vi "excelrowconcat.vi"() -> ()   [LabVIEW 2020]
uses:
  <vilib>/addons/_office/excel.llb/Excel Get Data ([dbl]).vi
  <vilib>/Utility/file.llb/Write To Spreadsheet File (DBL).vi
  <vilib>/Utility/NIReport.llb/NI_report.lvclass
  <vilib>/Utility/NIReport.llb/Excel/NI_Excel.lvclass
  <vilib>/addons/_office/NI_ReportGenerationToolkit.lvlib
panel:
  out "# Columns":i32
  out "# Rows":i32
  in  "Excel._Worksheet":refnum<k7>
  in  "Excel._Application":refnum<k7>
  out "Stack Col":ext[](array[numeric]) format="%#_6e"
  out "Selected Column":ext[](array[numeric])=[3.90764143958222e-05, 7.61822884669527e-05, 0.000114766080514528, 0.000154096182086505, 0.000194036736502312, 0.000211308521102183, 0.000244270893745124, 0.000280356936855242, 0.000316674588248134, 0.000346021261066198, 0.000431595311965793, 0.000475546228699386, 0.00051031302427873, 0.000549825024791062, 0.000611612165812403, 0.000633780786301941, 0.000619862112216651, 0.000508421915583313, 0.000282114429865032, 0.000305013061733916, 0.000323792832205072, 0.000337357050739229, 0.000354817893821746, 0.00036767779965885, 0.0004547196731437, 0.000476125016575679, 0.000460526207461953, 0.000503468560054898, 0.000534854829311371, 0.000561434135306627, 0.000575784360989928, 0.000602852320298553, 0.00058649032143876, 0.000528524222318083, 0.00047412229469046, 0.000426320446422324, 0.000394057540688664, 0.00035078008659184, 0.000306837755488232, 0.00027094132383354, 0.000238187931245193, 0.000209086530958302, 0.000183560623554513, 0.000159952367539518, 0.000138665272970684, 0.000119993324915413, 0.000103645805211272, 8.89317743713036e-05, 7.6019176049158e-05, 6.45195468678139e-05, 5.44001304660924e-05, 4.54942346550524e-05, 3.67294742318336e-05, 3.00935225823196e-05, 2.41571360675152e-05, 1.92496518138796e-05, 1.50192872752086e-05, 1.14403846964706e-05, 8.30091448733583e-06, 5.93545382798766e-06, 4.11274368161685e-06, 2.75384900305653e-06, 1.63597394475801e-06, 7.48674267470051e-07, 1.28115464903544e-08] format="%#_6e"
  in  "precission":string="6"
  in  "Destination path for cutting rows":path=path "C:/Users/lab user/Desktop/cm/New folder (2)"
  in  "row cut file name (no extension)":string="resultd9.xls"
  out "selected row":ext[](array[numeric])=[5.0, 14.0, 24.0, 34.887542] format="%#_6e"
  in  "Select Row Number (1,2,)":string="1,3,5"
  out "Total Selected Row":i32=3
  in  "Select Excel file":path=path "C:/Users/lab user/Desktop/cm/New folder (2)/D9.xls"
  out "Output Added row":ext[][](array[numeric])=[[1.0, 10.45566, 20.0, 30.0], [3.0, 12.0, 22.8765, 32.0], [5.0, 14.0, 24.0, 34.887542]] format="%#_6e"
  out "Sheet Values":ext[][](array[numeric])=[[1.0, 10.45566, 20.0, 30.0], [2.0, 11.0, 21.0, 31.0], [3.0, 12.0, 22.8765, 32.0], [4.0, 13.0, 23.0, 33.0], [5.0, 14.0, 24.0, 34.887542], [6.0, 15.0, 25.0, 35.0], [7.0, 16.0, 26.0, 36.0], [8.0, 17.0, 27.0, 37.0], [9.0, 18.0, 28.0, 38.0], [10.0, 19.0, 29.0, 39.0], [11.0, 20.0, 30.0, 40.0], [12.0, 21.0, 31.0, 41.0], [13.0, 22.0, 32.0, 42.0], [14.0, 23.0, 33.0, 43.0], [15.0, 24.0, 34.0, 44.0], [16.0, 25.0, 35.0, 45.0], [17.0, 26.0, 36.0, 46.0], [18.0, 27.0, 37.0, 47.0], [19.0, 28.0, 38.0, 48.0], [20.0, 29.0, 39.0, 49.0], [21.0, 30.0, 40.0, 50.0], [22.0, 31.0, 41.0, 51.0], [23.0, 32.0, 42.0, 52.0]] format="%_6e"
  # "_single column output will be save in same directory\nrow cut file name_single_col.xls"
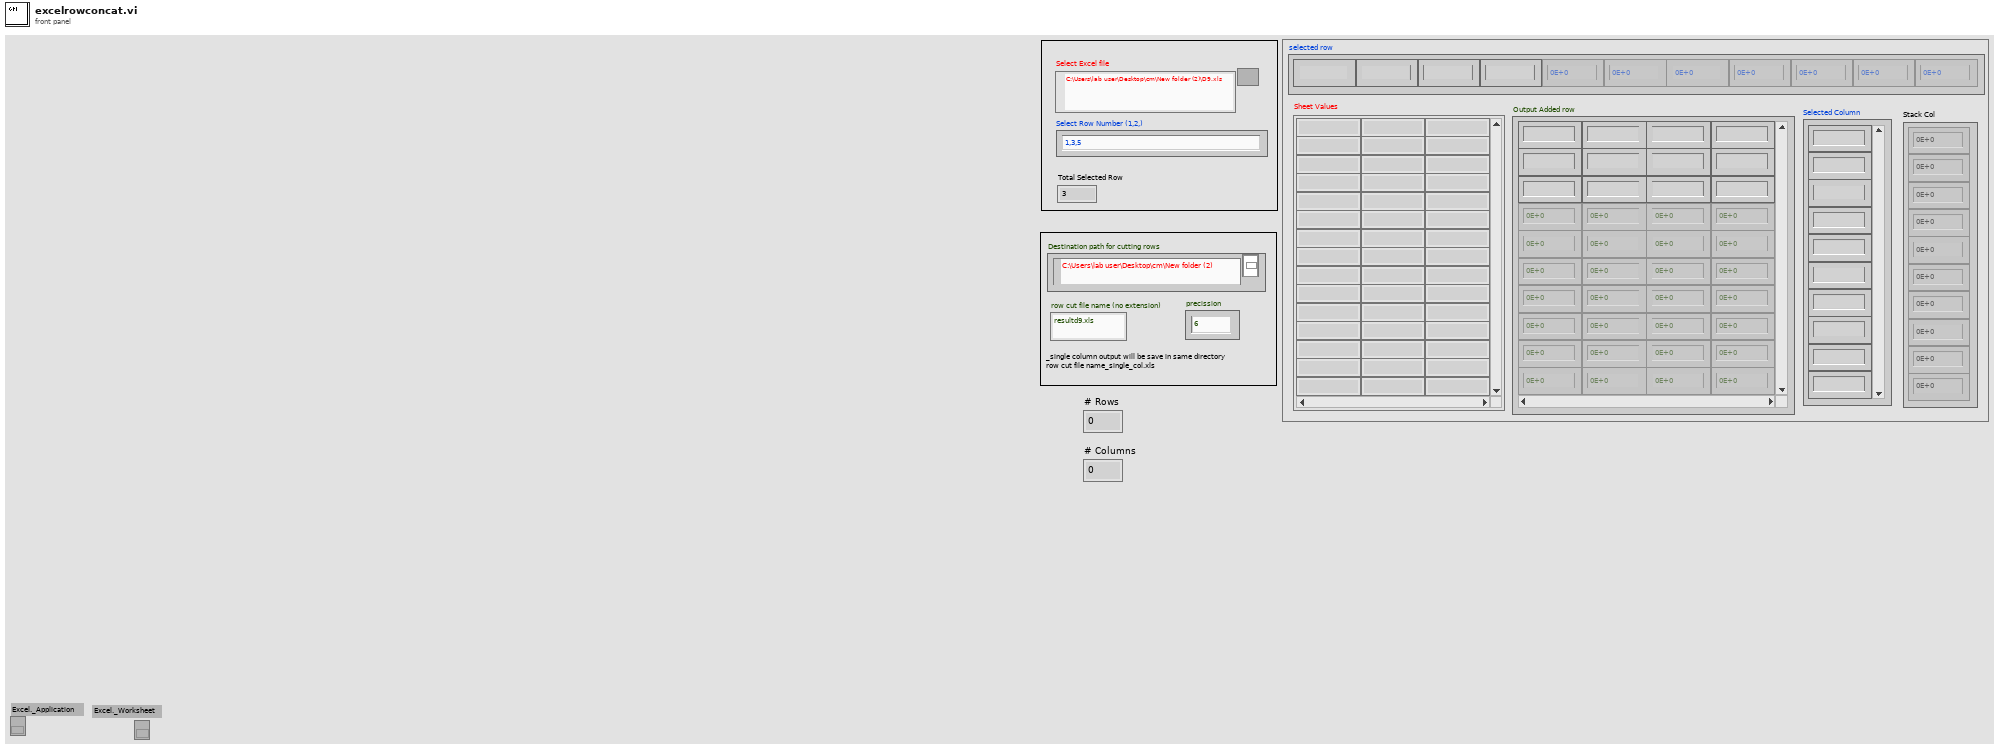
[diagram p1: front panel]
types:
  T1 = enum16{"Standard Report", "HTML", "Word", "Excel"}
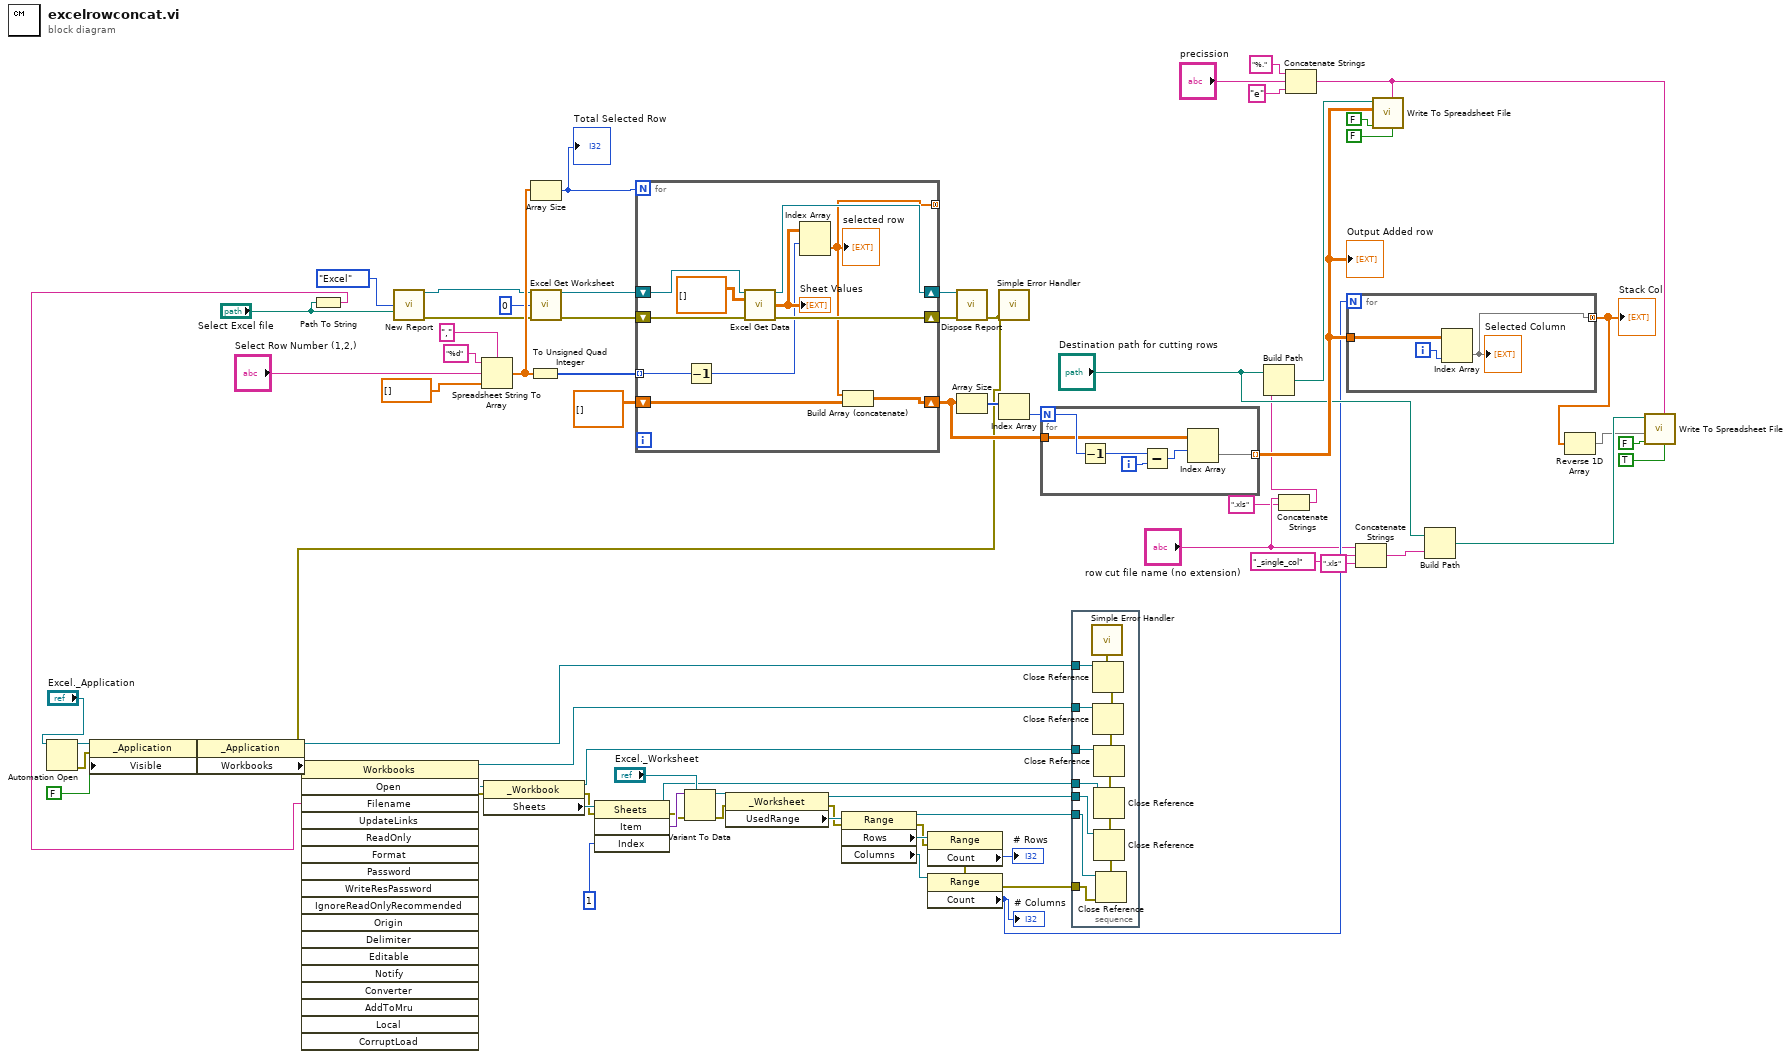
[diagram p0: block diagram]
diagram:
  n1 = Automation Open(Automation Refnum="Excel._Application") -> (Automation Refnum=w31:refnum<k7>, error out=w34:errorcluster)  [unwired: 3 in]
  n2 = property class="_Application"(reference=w31, error in=w34, "Visible"=FALSE ("Make Excel Visible")) -> (reference out=w30:refnum<k7>, error out=w33:errorcluster)
  n3 = property class="_Application"(reference=w30, error in=w33) -> (reference out=w16:refnum<k7>, "Workbooks"=w19:refnum<k7>)  [unwired: 1 out]
  n4 = Path To String(path="Select Excel file") -> (string=w8:string)
  n5 = call <vilib>:"New Report.vi"("report type"=T1."Excel", "template (empty)"="Select Excel file") -> ("report out"=w61:refnum<class "NI_report.lvclass">, "error out"=w62:errorcluster)  [unwired: 12 in]
  n6 = Spreadsheet String To Array(delimiter (Tab)=",", format string="%d", spreadsheet string="Select Row Number (1,2,)", array type (2D Dbl)=dbl[] []) -> (array=w65:dbl[])
  n7 = To Unsigned Quad Integer(1:w65) -> (0:w64:u64[])
  n8 = Array Size(array=w65) -> (size(s)=w41:i32)
  "Total Selected Row" <- w41
  n9 = call <vilib>:"Excel Get Worksheet.vi"("report in"=w61, "worksheet index (0)"=0, "error in (no error)"=w62) -> ("report out"=w59:refnum<class "NI_report.lvclass">, "error out"=w60:errorcluster)  [unwired: 11 in]
  n10 = for {
    N: w41 -> [_]
    shift-right: [w84] -> w74
    shift-left: w59 -> [w78]
    shift-right: [w83] -> w73
    shift-left: w60 -> [w79]
    shift-right: [w80] -> w58
    shift-left: ext[][] [] -> [w81]
    tunnel: w64 -> [w77] mode=indexing
    tunnel: [w75] -> _ mode=concatenating
    n11 = Decrement(x=w77) -> (x-1=w76:u64)
    n12 = call-poly <vilib>:"Excel Get Data.vi"("report in"=w78, "data type"=ext[][] [], "error in (no error)"=w79) -> ("report out"=w84:refnum<class "NI_report.lvclass">, "data"=w82:ext[][], "error out"=w83:errorcluster)  [unwired: 10 in]
    "Sheet Values" <- w82
    n13 = Index Array(array=w82, index (row)=w76) -> (element=w75:ext[])  [unwired: 1 in]
    "selected row" <- w75
    n14 = Build Array (concatenate)(w75, w81) -> (w80:ext[][])
  }
  n15 = call-dynamic "Dispose Report.vi"("report in"=w74, "error in (no error)"=w73) -> ("error out"=w7:errorcluster)  [unwired: 13 in]
  n16 = invoke class="Workbooks" method="Open"(reference=w19, error in=w7, "Filename"=w8) -> (reference out=w15:refnum<k7>, error out=w37:errorcluster, "Open"=w25:refnum<k7>)  [unwired: 15 in, 15 out]
  n17 = property class="_Workbook"(reference=w25, error in=w37) -> (reference out=w14:refnum<k7>, error out=w24:errorcluster, "Sheets"=w26:refnum<k7>)
  n18 = invoke class="Sheets" method="Item"(reference=w26, error in=w24, "Index"=1) -> (reference out=w13:refnum<k7>, error out=w23:errorcluster, "Item"=w36:variant)  [unwired: 1 in, 1 out]
  n19 = Variant To Data(error in=w23, type="Excel._Worksheet", Variant=w36) -> (data=w27:refnum<k7>, error out=w22:errorcluster)
  n20 = property class="_Worksheet"(reference=w27, error in=w22) -> (reference out=w12:refnum<k7>, error out=w21:errorcluster, "UsedRange"=w28:refnum<k7>)
  n21 = property class="Range"(reference=w28, error in=w21) -> (reference out=w11:refnum<k7>, error out=w20:errorcluster, "Rows"=w29:refnum<k7>, "Columns"=w17:refnum<k7>)
  n22 = property class="Range"(reference=w29, error in=w20) -> (error out=w10:errorcluster, "Count"=→"# Rows":i32)  [unwired: 1 out]
  n23 = property class="Range"(reference=w17, error in=w10) -> (error out=w9:errorcluster, "Count"=w6:i32)  [unwired: 1 out]
  "# Columns" <- w6
  n24 = Array Size(array=w58) -> (size(s)=w56:i32[])
  n25 = call <vilib>:"Simple Error Handler.vi"("error in (no error)"=w7) -> ()  [unwired: 4 in, 5 out]
  n26 = Index Array(array=w56) -> (element=w57:i32)  [unwired: 1 in]
  n27 = for {
    N: w57 -> [w91]
    tunnel: w58 -> [w88]
    tunnel: [w86] -> w49 mode=indexing
    i -> [w89]
    n28 = Decrement(x=w91) -> (x-1=w90:i32)
    n29 = Subtract(x=w90, y=w89) -> (x-y=w87:i32)
    n30 = Index Array(array=w88, index (row)=w87) -> (element=w86:ext[])  [unwired: 1 in]
  }
  "Output Added row" <- w49
  n31 = stacked-sequence {
    tunnel: w16 -> [w104]
    tunnel: w15 -> [w103]
    tunnel: w14 -> [w102]
    tunnel: w13 -> [w101]
    tunnel: w12 -> [w100]
    tunnel: w11 -> [w99]
    tunnel: w9 -> [w98]
    frame #0 {
      n32 = Close Reference(reference=w99, error in (no error)=w98) -> (error out=w97:errorcluster)
      n33 = Close Reference(reference=w100, error in (no error)=w97) -> (error out=w96:errorcluster)
      n34 = Close Reference(reference=w101, error in (no error)=w96) -> (error out=w95:errorcluster)
      n35 = Close Reference(reference=w102, error in (no error)=w95) -> (error out=w94:errorcluster)
      n36 = Close Reference(reference=w103, error in (no error)=w94) -> (error out=w93:errorcluster)
      n37 = Close Reference(reference=w104, error in (no error)=w93) -> (error out=w92:errorcluster)
      n38 = call <vilib>:"Simple Error Handler.vi"("error in (no error)"=w92) -> ()  [unwired: 4 in, 5 out]
    }
  }
  n39 = Concatenate Strings("row cut file name (no extension)", ".xls" ("string")) -> (w1:string)
  n40 = Build Path(base path="Destination path for cutting rows", name or relative path=w1) -> (appended path=w53:path)
  n41 = Concatenate Strings("%.", "precission", "e") -> (w42:string)
  n42 = for {
    N: w6 -> [_]
    tunnel: w49 -> [w106]
    tunnel: [w105] -> w40 mode=concatenating
    i -> [w107]
    n43 = Index Array(array=w106, index (col)=w107) -> (element=w105:ext[])  [unwired: 1 in]
    "Selected Column" <- w105
  }
  "Stack Col" <- w40
  n44 = Concatenate Strings("row cut file name (no extension)", "_single_col" ("string"), ".xls" ("string")) -> (w44:string)
  n45 = call-poly <vilib>:"Write To Spreadsheet File.vi"("transpose? (no:F)"=FALSE, "format (%.3f)"=w42, "append to file? (new file:F)"=FALSE, "2D data"=w49, "file path (dialog if empty)"=w53) -> ()  [unwired: 3 in, 1 out]
  n46 = Build Path(base path="Destination path for cutting rows", name or relative path=w44) -> (appended path=w46:path)
  n47 = Reverse 1D Array(array=w40) -> (reversed array=w39:ext[])
  n48 = call-poly <vilib>:"Write To Spreadsheet File.vi"("transpose? (no:F)"=TRUE, "format (%.3f)"=w42, "append to file? (new file:F)"=FALSE, "1D data"=w39, "file path (dialog if empty)"=w46) -> ()  [unwired: 3 in, 1 out]
